vi "BioFeedback22(v_0.3).vi"() -> ()   [LabVIEW 2016]
doc: "Use this template to build a producer/consumer design pattern. Use this template when you need to execute a process, such as data analysis, when a data source, such as a triggered acquisition, produces data at an uneven rate and you need to execute the process when the data becomes available."
uses:
  customSubVIs/8ChanWfmArray.ctl
  <vilib>/Utility/file.llb/Write Delimited Spreadsheet (string).vi
panel:
  in  "infiniteTrial":bool=TRUE caption="Infinite Trial"
  out "MVC State":enum16{"Nothing", "Saved MVC", "NoSave MVC"}(ring)
  in  "MVC Delay (s)":dbl=3.0
  out "trial last time":timestamp
  out "mvc last time":timestamp
  in  "Display Width for MVC (s)":dbl(slide)=1.0 caption="Window Width in Seconds" scale=0.1..10.0
  in  "Display Width for Current Trial":dbl(slide)=1.0 caption="Window Width in Seconds" scale=0.1..10.0
  out "Current Trial (Filtered)":waveform(dbl)(graph)
  out "Current MVC (Filtered)":waveform(dbl)(graph)
  in  "enableSave":bool=TRUE caption="No Save      Save"
  in  "barOrGraph":bool=TRUE caption="Graph (under construction)       Bar"
  in  "Trial comment":string
  out "Collecting Data":bool
  in  "Display Min":dbl
  in  "Display Max":dbl=100.0
  in  "log filepath":path
  out "TrialStartTime":timestamp
  in  "Trial Duration (s)":dbl=3.0
  out "Trial Number":dbl
  in  "Session Name":string="Default"
  out "loopTime":dbl=30.0 caption="Upper Cut-Off"
  in  "trial display data":path
  out "Disp Data":cluster{"queue out":refnum<queue>, dbl, dbl}[](array[cluster])
  in  "Target Percentage":dbl=10.0
  out "Current Activation":dbl
  out "DisplayBarActivation":dbl(slide) caption="Percent Activation" max=1.0 scale=0.0..100.0
  in  "EMG Channel To Display":dbl=1.0
  out "MVC Data":cluster{"queue out":refnum<queue>, dbl, dbl}[](array[cluster])
  out "Trial Name":string="Test"
  in  "Data Directory":path=path "C:/Users/Tinggroup/Desktop/EMG Biofeedback System/LabviewFiles/Data"
  out "GetMaxStartTime":timestamp
  in  "MVC Number":dbl=3.0
  in  "MVC Duration (s)":dbl=3.0
  in  "Frames Per Second":dbl=30.0 caption="Upper Cut-Off"
  in  "EMG Input Device\nProduct Type":string="USB-6009"
  out "raw data":dynamicdata(graph)
  out "dispSize":dbl=20.0 caption="Lower Cut-Off"
  out "mvcSize":dbl=300.0 caption="Upper Cut-Off"
  in  "MVC Window Size (s)":dbl=0.5
  in  "Display Window Size (s)":dbl=0.5
  in  "MVC Raw Path":path
  in  "trial raw data":path
  in  "trial filtered data":path
  in  "MVC Filtered Path":path
  in  "Sample rate (Hz)":dbl=1000.0 caption="Upper Cut-Off"
  out "fps":dbl=20.0 caption="Lower Cut-Off"
  out "rate":dbl=300.0 caption="Upper Cut-Off"
  in  "Set Parameters":bool
  out "lower":dbl=20.0 caption="Lower Cut-Off"
  out "upper":dbl=300.0 caption="Upper Cut-Off"
  in  "Lower Cut-Off":dbl=20.0
  in  "Upper Cut-Off":dbl=500.0
  in  "Mark":bool
  in  "End Trial":bool
  in  "Get MVC":bool
  in  "StartTrial":bool
  out "State":T1(ring)
  out "FilteredAndRectified":waveform(dbl)[](graph) caption="Filtered\nand\nRectified"
  in  "stop":bool
  # "Behind The Scenes"
  # "Add trial comment\nBEFORE beginning trial"
  # "Timing"
  # "Display Settings"
  # "Filtering"
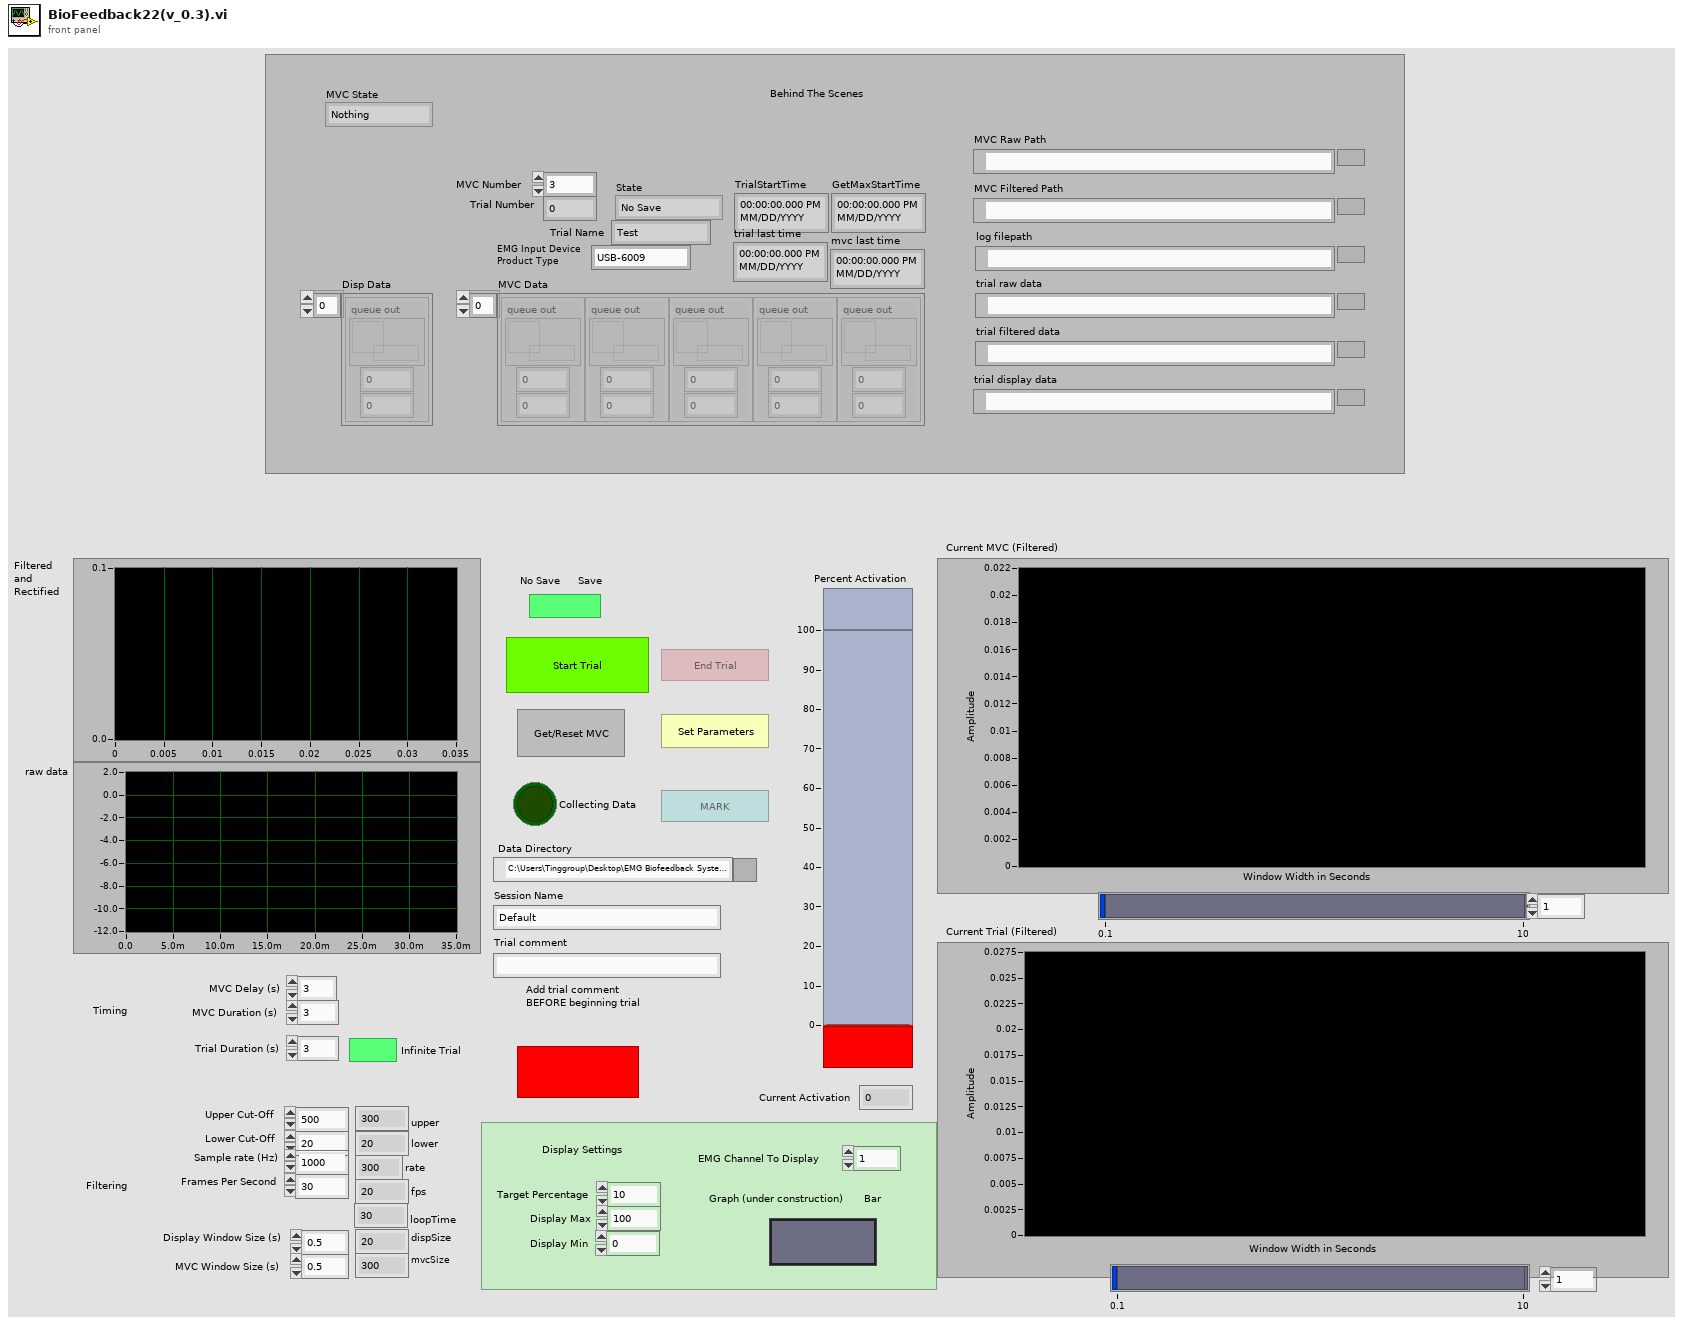
[diagram p1: front panel]
types:
  T1 = enum16{"No Save", "Acquiring Max", "Trial In Progress"}
  T2 = enum8{"Enabled", "Disabled", "Disabled and Grayed Out"}
  T3 = typedef "8ChanWfmArray.ctl" = waveform(dbl)[]
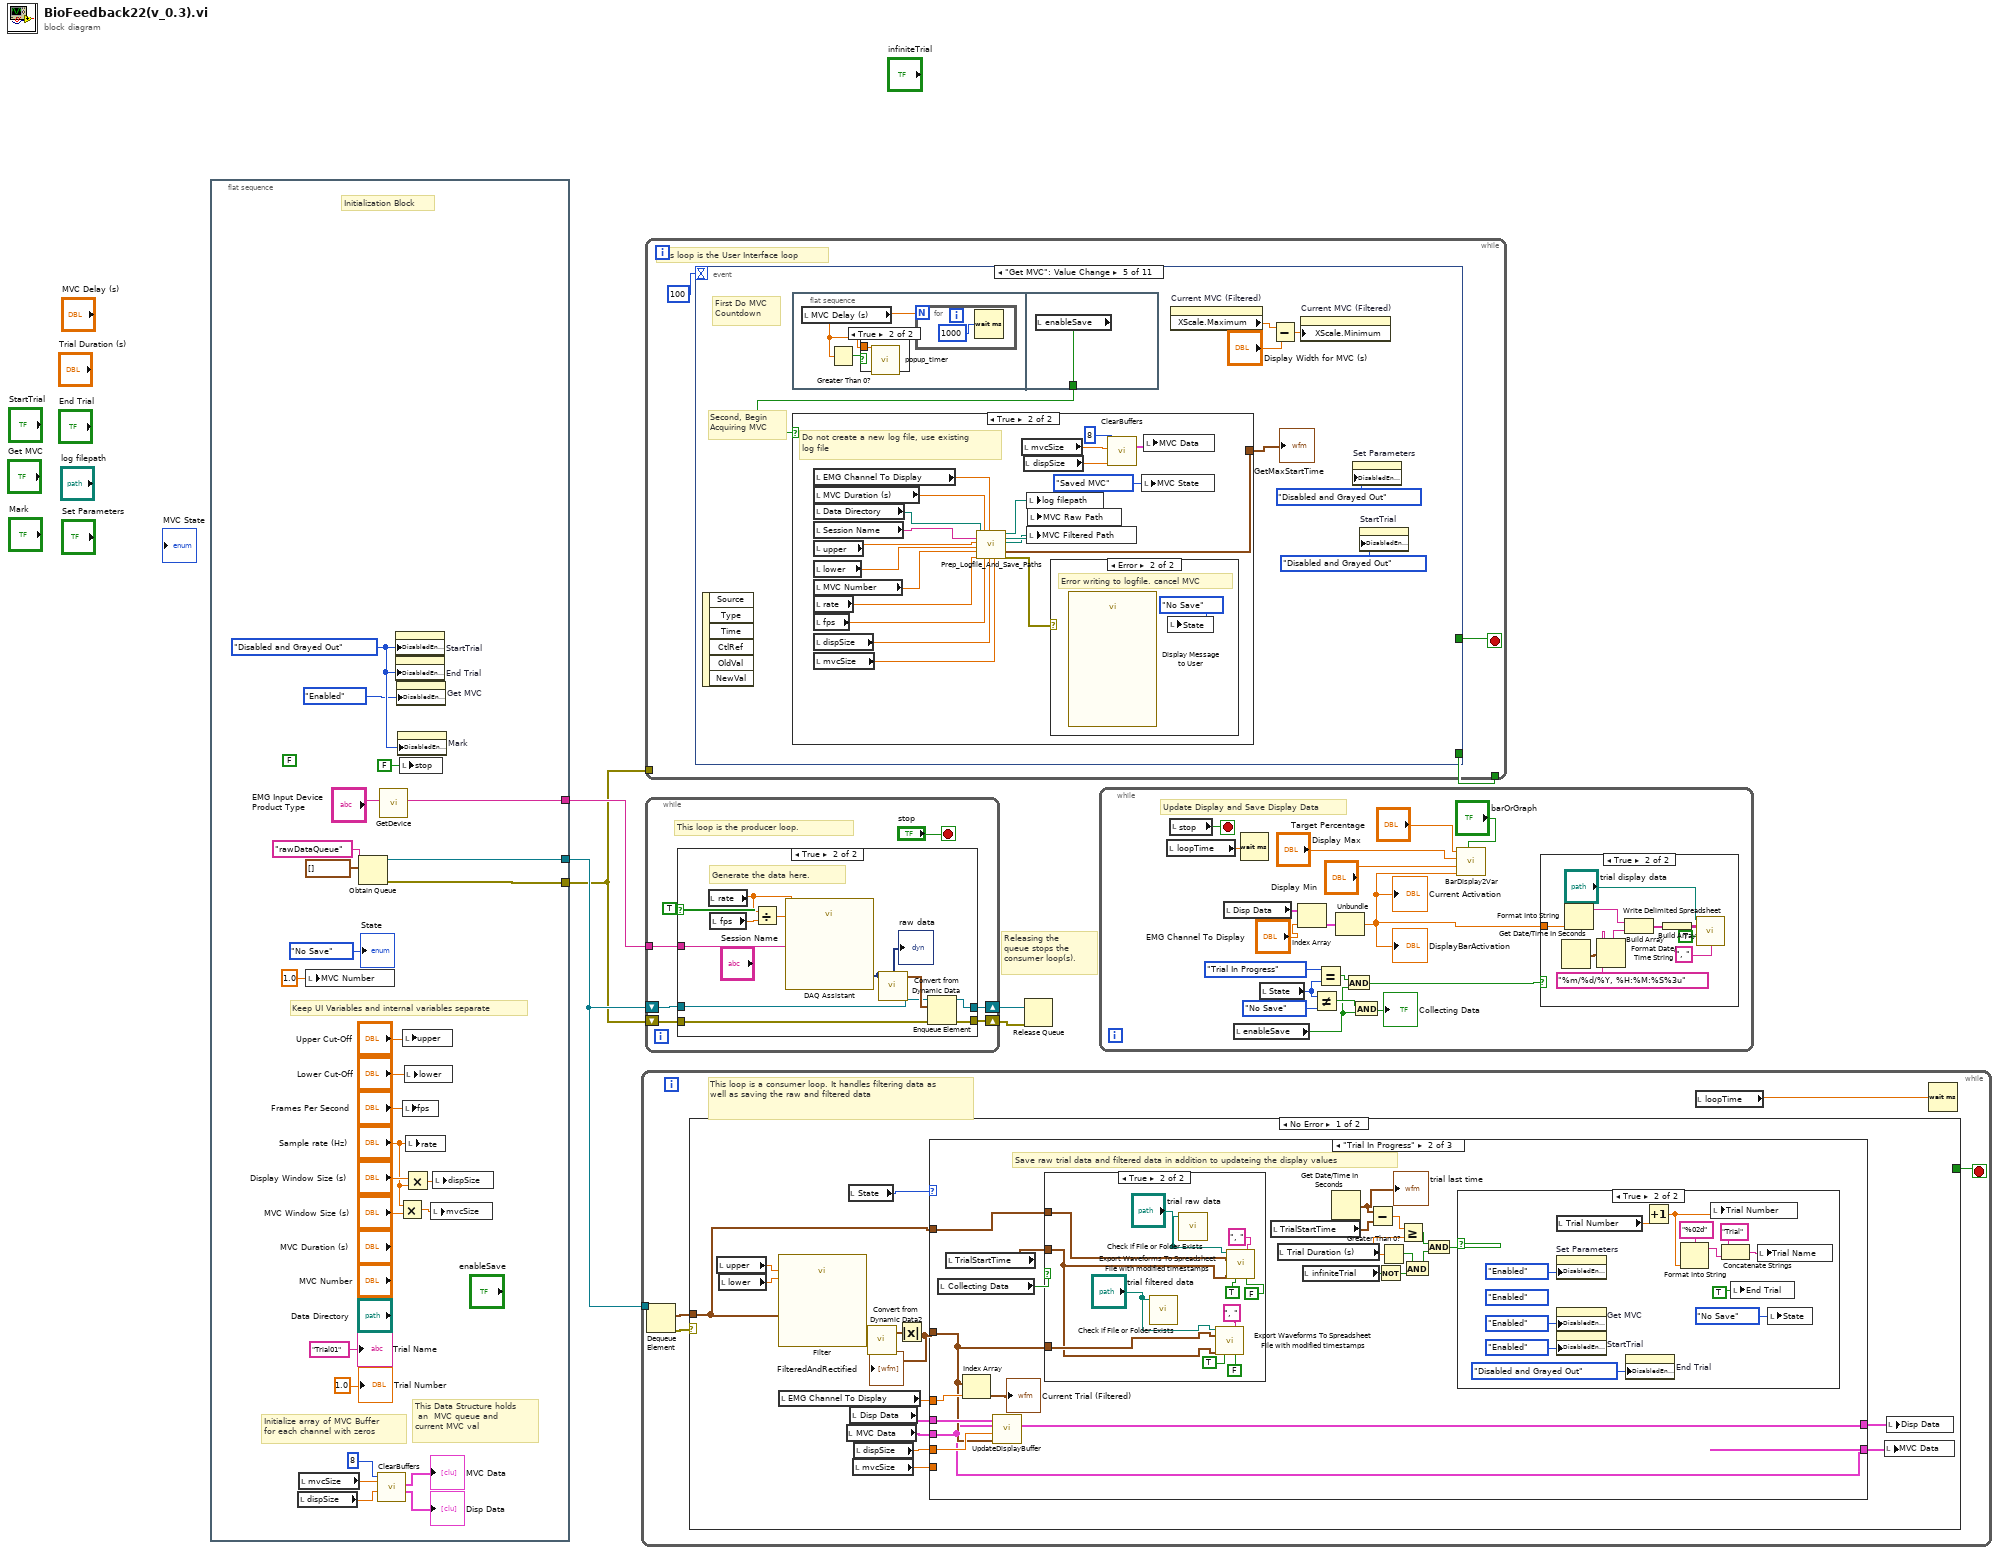
[diagram p0: block diagram]
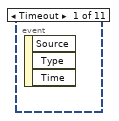
[diagram p3: hidden frame]
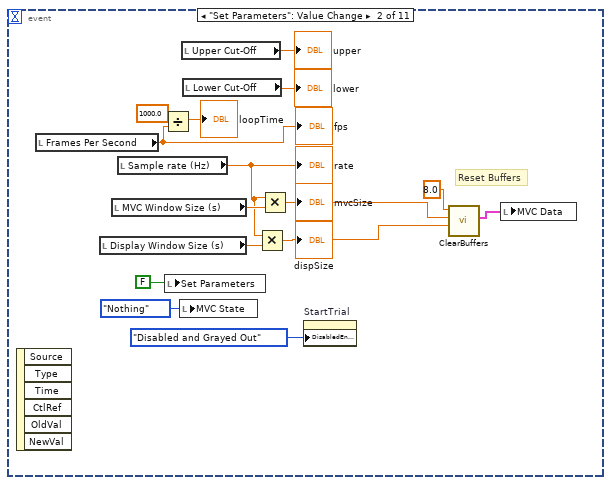
[diagram p4: hidden frame]
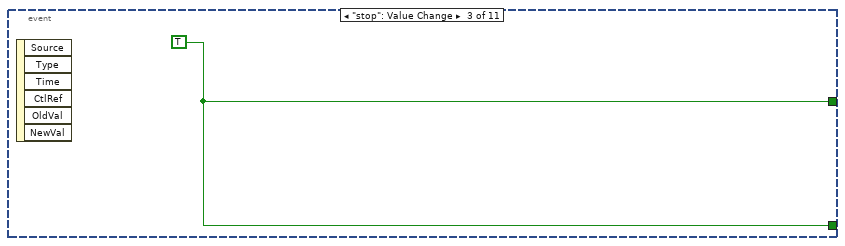
[diagram p5: hidden frame]
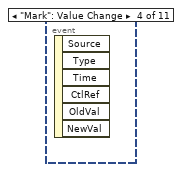
[diagram p6: hidden frame]
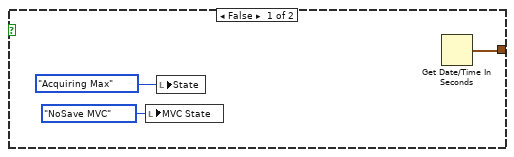
[diagram p8: hidden frame]
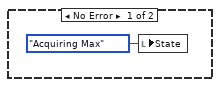
[diagram p9: hidden frame]
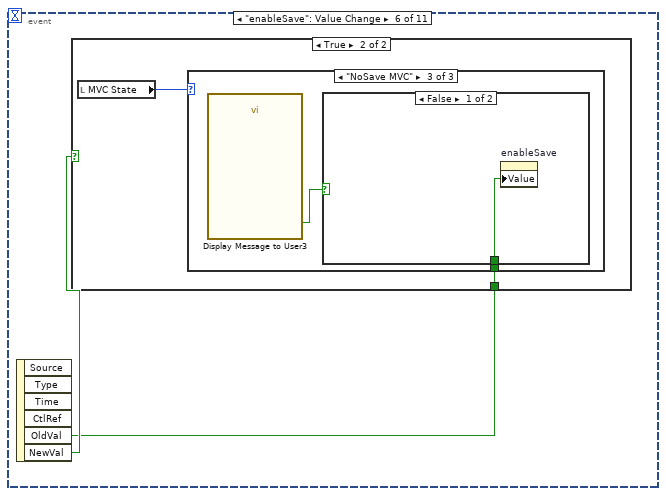
[diagram p10: hidden frame]
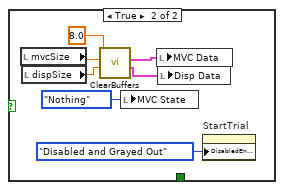
[diagram p14: hidden frame]
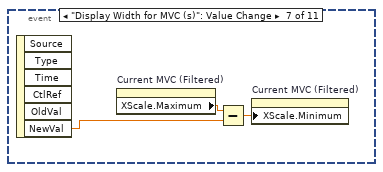
[diagram p15: hidden frame]
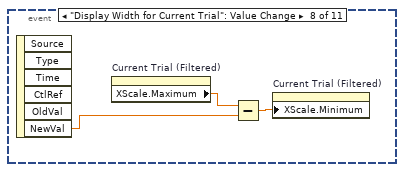
[diagram p16: hidden frame]
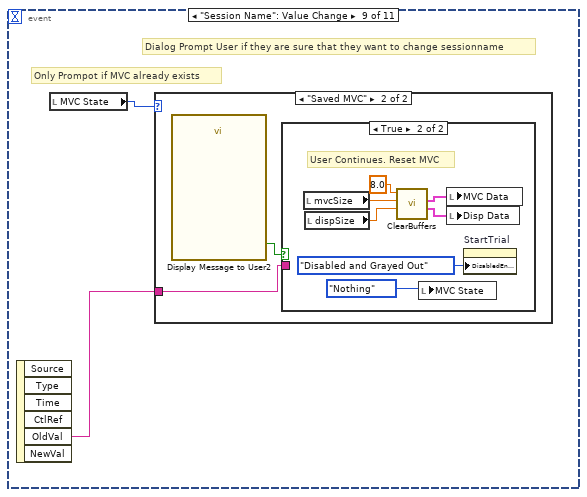
[diagram p17: hidden frame]
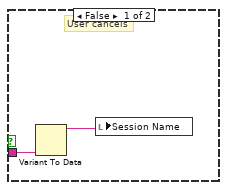
[diagram p19: hidden frame]
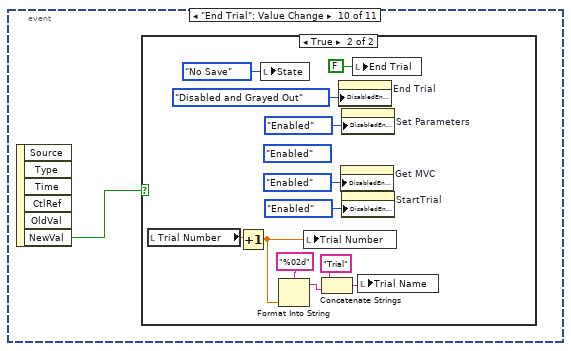
[diagram p20: hidden frame]
diagram:
  # "Releasing the\nqueue stops the consumer loop(s)."
  n1 = flat-sequence {
    tunnel: [w22] -> w2
    tunnel: [w21] -> w1
    tunnel: [w24] -> w3
    frame #0 {
      (unwired) FALSE ("Visible")
      w29 = T2."Disabled and Grayed Out" ("Disabled")
      # "Keep UI Variables and internal variables separate"
      # "This Data Structure holds\n an  MVC queue and \ncurrent MVC val"
      # "Initialize array of MVC Buffer \nfor each channel with zeros"
      # "Initialization Block"
      n2 = local read "dispSize"() -> (w9:dbl)
      n3 = local read "mvcSize"() -> (w10:dbl)
      n4 = local write "MVC Number"(1.0 ("MVC Number")) -> ()
      n5 = Obtain Queue(name (unnamed)="rawDataQueue", element data type=T3 [] ("initialized array")) -> (queue out=w22:refnum<queue>, error out=w21:errorcluster)  [unwired: 3 in, 1 out]
      n6 = call "ClearBuffers.vi"("disp size"=w9, "mvc size"=w10, "Num Channels"=8) -> ("Disp Data"=→"Disp Data":cluster{"queue out":refnum<queue>, dbl, dbl}[], "MVC Data"=→"MVC Data":cluster{"queue out":refnum<queue>, dbl, dbl}[])  [unwired: 7 in]
      n7 = call "GetDevice.vi"("EMG Input Device\nProduct Type"="EMG Input Device\nProduct Type") -> ("DAQmx Device Name"=w24:tag)  [unwired: 10 in]
      n8 = property on="StartTrial" class="Bool (strict)"("DisabledEnum"=w29) -> ()  [unwired: 2 in, 2 out]
      n9 = property on="End Trial" class="Bool (strict)"("DisabledEnum"=w29) -> ()  [unwired: 2 in, 2 out]
      n10 = property on="Get MVC" class="Bool"("DisabledEnum"=T2."Enabled" ("Disabled")) -> ()  [unwired: 2 in, 2 out]
      n11 = property on="Mark" class="Bool"("DisabledEnum"=w29) -> ()  [unwired: 2 in, 2 out]
      n12 = Multiply(x="Sample rate (Hz)", y="MVC Window Size (s)") -> (x*y=w16:dbl)
      n13 = local write "stop"(FALSE ("stop")) -> ()
      n14 = local write "upper"("Upper Cut-Off") -> ()
      n15 = local write "fps"("Frames Per Second") -> ()
      n16 = Multiply(x="Display Window Size (s)", y="Sample rate (Hz)") -> (x*y=w19:dbl)
      n17 = local write "lower"("Lower Cut-Off") -> ()
      n18 = local write "rate"("Sample rate (Hz)") -> ()
      n19 = local write "mvcSize"(w16) -> ()
      n20 = local write "dispSize"(w19) -> ()
      "Trial Name" <- "Trial01" ("Trial Name")
      "State" <- T1."No Save" ("State")
      "Trial Number" <- 1.0 ("Trial Number")
    }
  }
  n21 = while {
    tunnel: w2 -> [w33]
    stop <- w34 stop-if-true
    # "This loop is a consumer loop. It handles filtering data as well as saving the raw and filtered data"
    n22 = Dequeue Element(queue=w33) -> (element=w35:T3, error out=w36:errorcluster)  [unwired: 2 in, 2 out]
    n23 = case shown="No Error" w36 {
      tunnel: w35 -> [w46 _]
      tunnel: [_ TRUE] -> w34
      frame No Error {
        n24 = local read "upper"() -> (w48:dbl)
        n25 = local read "lower"() -> (w47:dbl)
        n26 = call "Filter"("Lower Cut-Off"=w47, "Upper Cut-Off"=w48, "Signal"=w46) -> ("Filtered Signal"=w49:dynamicdata)  [unwired: 7 in, 1 out]
        n27 = local read "EMG Channel To Display"() -> (w39:dbl)
        n28 = local read "MVC Data"() -> (w44:cluster{"queue out":refnum<queue>, dbl, dbl}[])
        n29 = local read "State"() -> (w40:T1)
        n30 = local read "Disp Data"() -> (w43:cluster{"queue out":refnum<queue>, dbl, dbl}[])
        n31 = local read "mvcSize"() -> (w37:dbl)
        n32 = local read "dispSize"() -> (w38:dbl)
        n33 = call "Convert from Dynamic Data2"("Dynamic Data Type"=w49) -> ("Array of Waveform"=w50:waveform(dbl)[])  [unwired: 3 in]
        n34 = Absolute Value(x=w50) -> (abs(x)=w45:waveform(dbl)[])
        "FilteredAndRectified" <- w45
        n35 = case shown="\"Trial In Progress\"" w40 {
          tunnel: w45 -> [w52 w61 w101]
          tunnel: w46 -> [_ w70 w110]
          tunnel: w44 -> [w54 w60 w104]
          tunnel: w43 -> [w55 w64 w105]
          tunnel: [w51 w62 w100] -> w41
          tunnel: [w54 w60 w99] -> w42
          tunnel: w39 -> [_ w67 w108]
          tunnel: w38 -> [w53 w63 w103]
          tunnel: w37 -> [_ _ w102]
          frame "No Save", Default {
            # "Update the display values, but do not save anything\n\nNote: MVC data is just referenced to calculate percent activation"
            n36 = call "UpdateDisplayBuffer.vi"("FilteredAndRectified"=w52, "dispSize"=w53, "MVC Data"=w54, "Disp Data"=w55) -> ("Disp Data Out"=w51:cluster{"queue out":refnum<queue>, dbl, dbl}[])  [unwired: 7 in]
          }
          frame "Trial In Progress" {
            # "Save raw trial data and filtered data in addition to updateing the display values"
            n37 = local read "Collecting Data"() -> (w69:bool)
            n38 = local read "TrialStartTime"() -> (w68:timestamp)
            n39 = Index Array(array=w61, index=w67) -> (element=→"Current Trial (Filtered)":waveform(dbl))
            n40 = call "UpdateDisplayBuffer.vi"("FilteredAndRectified"=w61, "dispSize"=w63, "MVC Data"=w60, "Disp Data"=w64) -> ("Disp Data Out"=w62:cluster{"queue out":refnum<queue>, dbl, dbl}[])  [unwired: 7 in]
            n41 = case shown="True" w69 {
              tunnel: w61 -> [_ w84]
              tunnel: w70 -> [_ w78]
              tunnel: w68 -> [_ w79]
              frame False {
              }
              frame True {
                n42 = call <vilib>:"Check if File or Folder Exists.vi"("path"="trial filtered data") -> ()  [unwired: 8 in, 3 out]
                n43 = call <vilib>:"Check if File or Folder Exists.vi"("path"="trial raw data") -> ()  [unwired: 8 in, 3 out]
                n44 = call "Export Waveforms To Spreadsheet File with modified timestamps.vi"("file path (dialog if empty)"="trial filtered data", "delimiter (Tab)"=", ", "waveforms"=w84, "trial start time"=w79, "append to file? (new file:F)"=TRUE, "header? (write header:T)"=FALSE) -> ()  [unwired: 8 in, 2 out]
                n45 = call "Export Waveforms To Spreadsheet File with modified timestamps.vi"("file path (dialog if empty)"="trial raw data", "delimiter (Tab)"=", ", "waveforms"=w78, "trial start time"=w79, "append to file? (new file:F)"=TRUE, "header? (write header:T)"=FALSE) -> ()  [unwired: 8 in, 2 out]
              }
            }
            n46 = local read "TrialStartTime"() -> (w74:timestamp)
            n47 = local read "Trial Duration (s)"() -> (w72:dbl)
            n48 = local read "infiniteTrial"() -> (w56:bool)
            n49 = Get Date/Time In Seconds() -> (seconds since 1Jan1904=w65:timestamp)
            "trial last time" <- w65
            n50 = Subtract(x=w65, y=w74) -> (x-y=w75:dbl)
            n51 = Not(x=w56) -> (.not. x?=w59:bool)
            n52 = Greater Than 0?(x=w72) -> (x > 0?=w58:bool)
            n53 = Greater Or Equal?(x=w75, y=w72) -> (x >= y?=w71:bool)
            n54 = And(x=w58, y=w59) -> (x .and. y?=w57:bool)
            n55 = And(x=w71, y=w57) -> (x .and. y?=w73:bool)
            n56 = case shown="True" w73 {
              frame False {
              }
              frame True {
                (unwired) T2."Enabled" ("Disabled")
                n57 = local read "Trial Number"() -> (w88:dbl)
                n58 = property on="Set Parameters" class="Bool (strict)"("DisabledEnum"=T2."Enabled" ("Disabled")) -> ()  [unwired: 2 in, 2 out]
                n59 = property on="Get MVC" class="Bool"("DisabledEnum"=T2."Enabled" ("Disabled")) -> ()  [unwired: 2 in, 2 out]
                n60 = property on="StartTrial" class="Bool (strict)"("DisabledEnum"=T2."Enabled" ("Disabled")) -> ()  [unwired: 2 in, 2 out]
                n61 = property on="End Trial" class="Bool (strict)"("DisabledEnum"=T2."Disabled and Grayed Out" ("Disabled")) -> ()  [unwired: 2 in, 2 out]
                n62 = Increment(x=w88) -> (x+1=w87:dbl)
                n63 = Format Into String(format string="%02d", w87) -> (resulting string=w93:string)  [unwired: 2 in, 1 out]
                n64 = local write "Trial Number"(w87) -> ()
                n65 = Concatenate Strings("Trial" ("string"), w93) -> (w97:string)
                n66 = local write "End Trial"(TRUE ("End Trial")) -> ()
                n67 = local write "Trial Name"(w97) -> ()
                n68 = local write "State"(T1."No Save" ("State")) -> ()
              }
            }
          }
          frame "Acquiring Max" {
            # "Automatically Stop Listening for Max after Acquire Max Time is elapsed"
            n69 = local read "GetMaxStartTime"() -> (w109:timestamp)
            n70 = local read "Collecting Data"() -> (w111:bool)
            n71 = call "UpdateMovingAverages.vi"("FilteredAndRectified"=w101, "mvcSize"=w102, "dispSize"=w103, "MVC Data"=w104, "Disp Data"=w105) -> ("MVC Data Out"=w99:cluster{"queue out":refnum<queue>, dbl, dbl}[], "Disp Data Out"=w100:cluster{"queue out":refnum<queue>, dbl, dbl}[])  [unwired: 5 in]
            n72 = case shown="True" w111 {
              tunnel: w110 -> [_ w118]
              tunnel: w101 -> [_ w124]
              tunnel: w109 -> [_ w119]
              frame False {
              }
              frame True {
                n73 = call "Export Waveforms To Spreadsheet File with modified timestamps.vi"("file path (dialog if empty)"="MVC Filtered Path", "delimiter (Tab)"=", ", "waveforms"=w124, "trial start time"=w119, "append to file? (new file:F)"=TRUE, "header? (write header:T)"=FALSE) -> ()  [unwired: 8 in, 2 out]
                n74 = call "Export Waveforms To Spreadsheet File with modified timestamps.vi"("file path (dialog if empty)"="MVC Raw Path", "delimiter (Tab)"=", ", "waveforms"=w118, "trial start time"=w119, "append to file? (new file:F)"=TRUE, "header? (write header:T)"=FALSE) -> ()  [unwired: 8 in, 2 out]
              }
            }
            n75 = Index Array(array=w101, index=w108) -> (element=→"Current MVC (Filtered)":waveform(dbl))
            n76 = local read "GetMaxStartTime"() -> (w115:timestamp)
            n77 = local read "MVC Duration (s)"() -> (w113:dbl)
            n78 = Get Date/Time In Seconds() -> (seconds since 1Jan1904=w106:timestamp)
            "mvc last time" <- w106
            n79 = Subtract(x=w106, y=w115) -> (x-y=w114:dbl)
            n80 = Greater Or Equal?(x=w114, y=w113) -> (x >= y?=w112:bool)
            n81 = case shown="True" w112 {
              frame False {
              }
              frame True {
                w128 = T2."Enabled" ("Disabled")
                n82 = local read "Collecting Data"() -> (w127:bool)
                n83 = local write "State"(T1."No Save" ("State")) -> ()
                n84 = property on="StartTrial" class="Bool (strict)"("DisabledEnum"=w128) -> ()  [unwired: 2 in, 2 out]
                n85 = property on="Set Parameters" class="Bool (strict)"("DisabledEnum"=w128) -> ()  [unwired: 2 in, 2 out]
                n86 = case shown="True" w127 {
                  frame False {
                  }
                  frame True {
                    n87 = local read "MVC Number"() -> (w131:dbl)
                    n88 = Increment(x=w131) -> (x+1=w130:dbl)
                    n89 = local write "MVC Number"(w130) -> ()
                  }
                }
              }
            }
          }
        }
        n90 = local write "MVC Data"(w42) -> ()
        n91 = local write "Disp Data"(w41) -> ()
      }
      frame Error {
        # "Return true for any case which should stop the loop."
      }
    }
    n92 = local read "loopTime"() -> (w32:dbl)
    n93 = Wait (ms)(milliseconds to wait=w32) -> ()  [unwired: 1 out]
  }
  n94 = while {
    tunnel: [w134] -> _
    tunnel: w1 -> [_]
    stop <- w133 stop-if-true
    # "This loop is the User Interface loop"
    n95 = event shown="[4] \"Get MVC\": Value Change" {
      selector: _ -> [_ _ _ _ _ _ _ _ _ _ _]
      dyn-events: _ -> [_ _ _ _ _ _ _ _ _ _ _]
      timeout: u32 100 ("milliseconds to wait") -> [_ _ _ _ _ _ _ _ _ _ _]
      tunnel: [_ _ w151 _ _ _ _ _ _ _ _] -> w133
      tunnel: [_ _ w151 _ _ _ _ _ _ _ _] -> w134
      event Timeout {
        n96 = event-data() -> ()  [unwired: 1 in, 3 out]
      }
      event "Set Parameters": Value Change {
        # "Reset Buffers"
        n97 = event-data() -> ()  [unwired: 1 in, 6 out]
        n98 = local read "Frames Per Second"() -> (w143:dbl)
        "fps" <- w143
        n99 = local read "Display Window Size (s)"() -> (w148:dbl)
        n100 = local read "MVC Window Size (s)"() -> (w149:dbl)
        n101 = local read "Sample rate (Hz)"() -> (w146:dbl)
        "rate" <- w146
        n102 = Divide(x=1000.0, y=w143) -> (x/y=→"loopTime":dbl)
        n103 = local write "Set Parameters"(FALSE ("Set Parameters")) -> ()
        n104 = local write "MVC State"(enum16{"Nothing", "Saved MVC", "NoSave MVC"}."Nothing" ("MVC State")) -> ()
        n105 = local read "Upper Cut-Off"() -> (→"upper":dbl)
        n106 = local read "Lower Cut-Off"() -> (→"lower":dbl)
        n107 = Multiply(x=w146, y=w148) -> (x*y=w140:dbl)
        "dispSize" <- w140
        n108 = Multiply(x=w146, y=w149) -> (x*y=w141:dbl)
        "mvcSize" <- w141
        n109 = property on="StartTrial" class="Bool (strict)"("DisabledEnum"=T2."Disabled and Grayed Out" ("Disabled")) -> ()  [unwired: 2 in, 2 out]
        n110 = call "ClearBuffers.vi"("disp size"=w140, "mvc size"=w141, "Num Channels"=8.0) -> ("MVC Data"=w138:cluster{"queue out":refnum<queue>, dbl, dbl}[])  [unwired: 7 in, 1 out]
        n111 = local write "MVC Data"(w138) -> ()
      }
      event "stop": Value Change {
        w151 = TRUE
        n112 = event-data() -> ()  [unwired: 1 in, 6 out]
      }
      event "Mark": Value Change {
        n113 = event-data() -> ()  [unwired: 1 in, 6 out]
      }
      event "Get MVC": Value Change {
        # "Second, Begin \nAcquiring MVC"
        # "First Do MVC\nCountdown"
        n114 = event-data() -> ()  [unwired: 1 in, 6 out]
        n115 = flat-sequence {
          tunnel: [w163] -> w156
          frame #0 {
            n116 = local read "MVC Delay (s)"() -> (w159:dbl)
            n117 = Greater Than 0?(x=w159) -> (x > 0?=w160:bool)
            n118 = case shown="True" w160 {
              tunnel: w159 -> [_ w161]
              frame False {
              }
              frame True {
                n119 = call "popup_timer.vi"("Seconds"=w161) -> ()  [unwired: 9 in, 1 out]
              }
            }
            n120 = for {
              N: w159 -> [_]
              n121 = Wait (ms)(milliseconds to wait=u32 1000) -> ()  [unwired: 1 out]
            }
          }
          frame #1 {
            n122 = local read "enableSave"() -> (w163:bool)
          }
        }
        n123 = case shown="True" w156 {
          tunnel: [w164 w167] -> w154
          frame False {
            n124 = local write "MVC State"(enum16{"Nothing", "Saved MVC", "NoSave MVC"}."NoSave MVC" ("MVC State")) -> ()
            n125 = local write "State"(T1."Acquiring Max" ("State")) -> ()
            n126 = Get Date/Time In Seconds() -> (seconds since 1Jan1904=w164:timestamp)
          }
          frame True {
            # "Do not create a new log file, use existing \nlog file"
            n127 = local read "EMG Channel To Display"() -> (w170:dbl)
            n128 = local read "MVC Duration (s)"() -> (w171:dbl)
            n129 = local read "Data Directory"() -> (w183:path)
            n130 = local read "Session Name"() -> (w182:string)
            n131 = local read "upper"() -> (w179:dbl)
            n132 = local read "lower"() -> (w178:dbl)
            n133 = local read "MVC Number"() -> (w177:dbl)
            n134 = local read "rate"() -> (w175:dbl)
            n135 = local read "fps"() -> (w174:dbl)
            n136 = local read "dispSize"() -> (w173:dbl)
            n137 = local read "mvcSize"() -> (w172:dbl)
            n138 = call "Prep_Logfile_And_Save_Paths.vi"("Data Directory"=w183, "Session Name"=w182, "upper"=w179, "lower"=w178, "MVC Number"=w177, "rate"=w175, "MVC Duration (s)"=w171, "fps"=w174, "EMG Channel To Display"=w170, "dispSize"=w173, "mvcSize"=w172) -> ("log filepath"=w181:path, "MVC Raw Path"=w180:path, "MVC Filtered Path"=w176:path, "GetMaxStartTime"=w167:timestamp, "error out"=w169:errorcluster)  [unwired: 4 in]
            n139 = local read "mvcSize"() -> (w186:dbl)
            n140 = local read "dispSize"() -> (w184:dbl)
            n141 = local write "log filepath"(w181) -> ()
            n142 = local write "MVC Filtered Path"(w176) -> ()
            n143 = local write "MVC Raw Path"(w180) -> ()
            n144 = case shown="Error" w169 {
              frame No Error {
                n145 = local write "State"(T1."Acquiring Max" ("State")) -> ()
              }
              frame Error {
                # "Error writing to logfile. cancel MVC"
                n146 = call "Display Message to User"() -> ()  [unwired: 10 in, 2 out]
                n147 = local write "State"(T1."No Save" ("State")) -> ()
              }
            }
            n148 = call "ClearBuffers.vi"("disp size"=w184, "mvc size"=w186, "Num Channels"=8) -> ("MVC Data"=w187:cluster{"queue out":refnum<queue>, dbl, dbl}[])  [unwired: 7 in, 1 out]
            n149 = local write "MVC State"(enum16{"Nothing", "Saved MVC", "NoSave MVC"}."Saved MVC" ("MVC State")) -> ()
            n150 = local write "MVC Data"(w187) -> ()
          }
        }
        "GetMaxStartTime" <- w154
        n151 = property on="Current MVC (Filtered)" class="WFChart (strict)"() -> ("XScale.Maximum"=w152:dbl)  [unwired: 2 in, 2 out]
        n152 = Subtract(x=w152, y="Display Width for MVC (s)") -> (x-y=w155:dbl)
        n153 = property on="Current MVC (Filtered)" class="WFChart (strict)"("XScale.Minimum"=w155) -> ()  [unwired: 2 in, 2 out]
        n154 = property on="Set Parameters" class="Bool (strict)"("DisabledEnum"=T2."Disabled and Grayed Out" ("Disabled")) -> ()  [unwired: 2 in, 2 out]
        n155 = property on="StartTrial" class="Bool (strict)"("DisabledEnum"=T2."Disabled and Grayed Out" ("Disabled")) -> ()  [unwired: 2 in, 2 out]
      }
      event "enableSave": Value Change {
        n156 = event-data() -> ("OldVal"=w190:bool, "NewVal"=w191:bool)  [unwired: 1 in, 4 out]
        n157 = case shown="True" w191 {
          tunnel: w190 -> [_ w192]
          frame False {
          }
          frame True {
            n158 = local read "MVC State"() -> (w193:enum16{"Nothing", "Saved MVC", "NoSave MVC"})
            n159 = case shown="\"NoSave MVC\"" w193 {
              tunnel: w192 -> [_ _ w194]
              frame "Nothing", Default {
              }
              frame "Saved MVC" {
              }
              frame "NoSave MVC" {
                n160 = call "Display Message to User3"() -> ("Enable Saving"=w195:bool)  [unwired: 10 in, 1 out]
                n161 = case shown="False" w195 {
                  tunnel: w194 -> [w196 _]
                  frame False {
                    n162 = property on="enableSave" class="Bool (strict)"("Value"=w196) -> ()  [unwired: 2 in, 2 out]
                  }
                  frame True {
                    n163 = local read "mvcSize"() -> (w201:dbl)
                    n164 = local read "dispSize"() -> (w200:dbl)
                    n165 = call "ClearBuffers.vi"("disp size"=w200, "mvc size"=w201, "Num Channels"=8.0) -> ("Disp Data"=w203:cluster{"queue out":refnum<queue>, dbl, dbl}[], "MVC Data"=w202:cluster{"queue out":refnum<queue>, dbl, dbl}[])  [unwired: 7 in]
                    n166 = local write "MVC State"(enum16{"Nothing", "Saved MVC", "NoSave MVC"}."Nothing" ("MVC State")) -> ()
                    n167 = local write "MVC Data"(w202) -> ()
                    n168 = local write "Disp Data"(w203) -> ()
                    n169 = property on="StartTrial" class="Bool (strict)"("DisabledEnum"=T2."Disabled and Grayed Out" ("Disabled")) -> ()  [unwired: 2 in, 2 out]
                  }
                }
              }
            }
          }
        }
      }
      event "Display Width for MVC (s)": Value Change {
        n170 = event-data() -> ("NewVal"=w206:dbl)  [unwired: 1 in, 5 out]
        n171 = property on="Current MVC (Filtered)" class="WFChart (strict)"() -> ("XScale.Maximum"=w204:dbl)  [unwired: 2 in, 2 out]
        n172 = Subtract(x=w204, y=w206) -> (x-y=w205:dbl)
        n173 = property on="Current MVC (Filtered)" class="WFChart (strict)"("XScale.Minimum"=w205) -> ()  [unwired: 2 in, 2 out]
      }
      event "Display Width for Current Trial": Value Change {
        n174 = event-data() -> ("NewVal"=w209:dbl)  [unwired: 1 in, 5 out]
        n175 = property on="Current Trial (Filtered)" class="WFChart (strict)"() -> ("XScale.Maximum"=w207:dbl)  [unwired: 2 in, 2 out]
        n176 = Subtract(x=w207, y=w209) -> (x-y=w208:dbl)
        n177 = property on="Current Trial (Filtered)" class="WFChart (strict)"("XScale.Minimum"=w208) -> ()  [unwired: 2 in, 2 out]
      }
      event "Session Name": Value Change {
        # "Only Prompot if MVC already exists"
        # "Dialog Prompt User if they are sure that they want to change sessionname"
        n178 = event-data() -> ("OldVal"=w211:string)  [unwired: 1 in, 5 out]
        n179 = local read "MVC State"() -> (w210:enum16{"Nothing", "Saved MVC", "NoSave MVC"})
        n180 = case shown="\"Saved MVC\"" w210 {
          tunnel: w211 -> [_ w212]
          frame "Nothing", Default {
          }
          frame "Saved MVC" {
            n181 = call "Display Message to User2"() -> ("Change"=w213:bool)  [unwired: 10 in, 1 out]
            n182 = case shown="True" w213 {
              tunnel: w212 -> [w215 _]
              frame False {
                # "User cancels"
                n183 = Variant To Data(Variant=w215) -> (data=w214:string)  [unwired: 2 in, 1 out]
                n184 = local write "Session Name"(w214) -> ()
              }
              frame True {
                # "User Continues. Reset MVC"
                n185 = local read "mvcSize"() -> (w221:dbl)
                n186 = local read "dispSize"() -> (w220:dbl)
                n187 = call "ClearBuffers.vi"("disp size"=w220, "mvc size"=w221, "Num Channels"=8.0) -> ("Disp Data"=w217:cluster{"queue out":refnum<queue>, dbl, dbl}[], "MVC Data"=w218:cluster{"queue out":refnum<queue>, dbl, dbl}[])  [unwired: 7 in]
                n188 = local write "MVC State"(enum16{"Nothing", "Saved MVC", "NoSave MVC"}."Nothing" ("MVC State")) -> ()
                n189 = local write "MVC Data"(w218) -> ()
                n190 = local write "Disp Data"(w217) -> ()
                n191 = property on="StartTrial" class="Bool (strict)"("DisabledEnum"=T2."Disabled and Grayed Out" ("Disabled")) -> ()  [unwired: 2 in, 2 out]
              }
            }
          }
        }
      }
      event "End Trial": Value Change {
        n192 = event-data() -> ("NewVal"=w223:bool)  [unwired: 1 in, 5 out]
        n193 = case shown="True" w223 {
          frame False {
          }
          frame True {
            (unwired) T2."Enabled" ("Disabled")
            n194 = local read "Trial Number"() -> (w228:dbl)
            n195 = Increment(x=w228) -> (x+1=w224:dbl)
            n196 = local write "State"(T1."No Save" ("State")) -> ()
            n197 = Format Into String(format string="%02d", w224) -> (resulting string=w227:string)  [unwired: 2 in, 1 out]
            n198 = local write "Trial Number"(w224) -> ()
            n199 = Concatenate Strings("Trial" ("string"), w227) -> (w229:string)
            n200 = property on="End Trial" class="Bool (strict)"("DisabledEnum"=T2."Disabled and Grayed Out" ("Disabled")) -> ()  [unwired: 2 in, 2 out]
            n201 = property on="Get MVC" class="Bool"("DisabledEnum"=T2."Enabled" ("Disabled")) -> ()  [unwired: 2 in, 2 out]
            n202 = property on="Set Parameters" class="Bool (strict)"("DisabledEnum"=T2."Enabled" ("Disabled")) -> ()  [unwired: 2 in, 2 out]
            n203 = property on="StartTrial" class="Bool (strict)"("DisabledEnum"=T2."Enabled" ("Disabled")) -> ()  [unwired: 2 in, 2 out]
            n204 = local write "End Trial"(FALSE ("End Trial")) -> ()
            n205 = local write "Trial Name"(w229) -> ()
          }
        }
      }
      event "StartTrial": Value Change {
        n206 = event-data() -> ("NewVal"=w236:bool)  [unwired: 1 in, 5 out]
        n207 = case shown="True" w236 {
          frame False {
          }
          frame True {
            (unwired) T2."Disabled and Grayed Out" ("Disabled")
            n208 = local write "StartTrial"(FALSE ("StartTrial")) -> ()
            n209 = local read "Data Directory"() -> (w284:path)
            n210 = local write "End Trial"(FALSE ("End Trial")) -> ()
            n211 = local read "Session Name"() -> (w283:string)
            n212 = local read "Trial Name"() -> (w268:string)
            n213 = local write "State"(T1."Trial In Progress" ("State")) -> ()
            n214 = Concatenate Strings(w268, "_FilteredData.csv" ("string")) -> (w288:string)
            n215 = Concatenate Strings(w268, "_RawData.csv" ("string")) -> (w286:string)
            n216 = Concatenate Strings(w268, "_DisplayData.csv" ("string")) -> (w290:string)
            n217 = property on="Current Trial (Filtered)" class="WFChart (strict)"() -> ("XScale.Maximum"=w237:dbl)  [unwired: 2 in, 2 out]
            n218 = Build Path(base path=w284, name or relative path=w283) -> (appended path=w267:path)
            n219 = property on="End Trial" class="Bool (strict)"("DisabledEnum"=T2."Enabled" ("Disabled")) -> ()  [unwired: 2 in, 2 out]
            n220 = property on="StartTrial" class="Bool (strict)"("DisabledEnum"=T2."Disabled and Grayed Out" ("Disabled")) -> ()  [unwired: 2 in, 2 out]
            n221 = property on="Get MVC" class="Bool"("DisabledEnum"=T2."Disabled and Grayed Out" ("Disabled")) -> ()  [unwired: 2 in, 2 out]
            n222 = property on="Set Parameters" class="Bool (strict)"("DisabledEnum"=T2."Disabled and Grayed Out" ("Disabled")) -> ()  [unwired: 2 in, 2 out]
            n223 = Build Path(base path=w267, name or relative path="Log.csv" ("string")) -> (appended path=w251:path)
            n224 = Build Path(base path=w267, name or relative path=w288) -> (appended path=w282:path)
            n225 = Build Path(base path=w267, name or relative path=w286) -> (appended path=w281:path)
            n226 = Build Path(base path=w267, name or relative path=w290) -> (appended path=w291:path)
            n227 = Get Date/Time In Seconds() -> (seconds since 1Jan1904=→"TrialStartTime":timestamp)
            n228 = local write "trial raw data"(w281) -> ()
            n229 = local write "log filepath"(w251) -> ()
            n230 = local write "trial filtered data"(w282) -> ()
            n231 = local write "trial display data"(w291) -> ()
            n232 = Subtract(x=w237, y="Display Width for Current Trial") -> (x-y=w240:dbl)
            n233 = property on="Current MVC (Filtered)" class="WFChart (strict)"("XScale.Minimum"=w240) -> ()  [unwired: 2 in, 2 out]
            n234 = local read "EMG Channel To Display"() -> (w247:dbl)
            n235 = local read "EMG Channel To Display"() -> (w277:dbl)
            n236 = local read "MVC Data"() -> (w248:cluster{"queue out":refnum<queue>, dbl, dbl}[])
            n237 = local read "MVC Duration (s)"() -> (w276:dbl)
            n238 = local read "dispSize"() -> (w274:dbl)
            n239 = local read "lower"() -> (w271:dbl)
            n240 = Index Array(array=w248, index=w247) -> (element=w246:cluster{"queue out":refnum<queue>, dbl, dbl})
            n241 = local read "mvcSize"() -> (w275:dbl)
            n242 = local read "upper"() -> (w270:dbl)
            n243 = local read "Trial Name"() -> (w264:string)
            n244 = local read "rate"() -> (w272:dbl)
            n245 = local read "fps"() -> (w273:dbl)
            n246 = Number To Decimal String(number=w271) -> (decimal integer string=w260:string)  [unwired: 1 in]
            n247 = Number To Decimal String(number=w274) -> (decimal integer string=w258:string)  [unwired: 1 in]
            n248 = Unbundle(w246) -> (w242:dbl)  [unwired: 2 out]
            n249 = Number To Decimal String(number=w277) -> (decimal integer string=w255:string)  [unwired: 1 in]
            n250 = Get Date/Time In Seconds() -> (seconds since 1Jan1904=w250:timestamp)
            n251 = Number To Decimal String(number=w270) -> (decimal integer string=w261:string)  [unwired: 1 in]
            n252 = Number To Decimal String(number=w272) -> (decimal integer string=w259:string)  [unwired: 1 in]
            n253 = Number To Decimal String(number=w273) -> (decimal integer string=w254:string)  [unwired: 1 in]
            n254 = Number To Decimal String(number=w275) -> (decimal integer string=w257:string)  [unwired: 1 in]
            n255 = Number To Decimal String(number=w276) -> (decimal integer string=w256:string)  [unwired: 1 in]
            n256 = Format Date/Time String(time format string (%c)="%m/%d/%Y %H:%M:%S%3u", seconds (now)=w250) -> (date/time string=w245:string)  [unwired: 1 in]
            n257 = Format Value(format string="%5f", value (0)=w242) -> (output string=w241:string)  [unwired: 1 in]
            n258 = Build Array(w264, w261, w260, w259, w254, w258, w257, w256, w255, w241, w245, "Trial comment") -> (w253:string[])
            n259 = call-poly <vilib>:"Write Delimited Spreadsheet.vi"("file path (dialog if empty)"=w251, "1D data"=w253, "append to file? (new file:F)"=TRUE, "delimiter (\\t)"=", " ("delimiter (\\t)")) -> ()  [unwired: 10 in, 2 out]
          }
        }
      }
    }
  }
  n260 = while {
    shift-right: [w296] -> w4
    shift-left: w1 -> [w297]
    shift-right: [w293] -> w5
    shift-left: w2 -> [w298]
    tunnel: w3 -> [w294]
    stop <- "stop" stop-if-true
    # "This loop is the producer loop."
    n261 = case shown="True" TRUE ("Case Constant\n(See Context Help)") {
      tunnel: w298 -> [w300 w303]
      tunnel: w297 -> [w301 w311]
      tunnel: [w301 w310] -> w296
      tunnel: w294 -> [_ w305]
      tunnel: [w300 w302] -> w293
      frame False {
      }
      frame True {
        # "Generate the data here."
        n262 = local read "rate"() -> (w308:dbl)
        n263 = local read "fps"() -> (w309:dbl)
        n264 = Divide(x=w308, y=w309) -> (x/y=w307:dbl)
        n265 = call "DAQ Assistant"("rate"=w308, "number of samples"=w307, "device name"=w305) -> ("data"=w306:dynamicdata)  [unwired: 13 in, 3 out]
        "raw data" <- w306
        n266 = call "Convert from Dynamic Data"("Dynamic Data Type"=w306) -> ("Array of Waveform"=w304:waveform(dbl)[])  [unwired: 3 in]
        n267 = Enqueue Element(queue=w303, element=w304, error in (no error)=w311) -> (queue out=w302:refnum<queue>, error out=w310:errorcluster)  [unwired: 1 in, 1 out]
      }
    }
  }
  n268 = Release Queue(queue=w5, error in (no error)=w4) -> ()  [unwired: 1 in, 3 out]
  n269 = while {
    stop <- w325 stop-if-true
    # "Update Display and Save Display Data"
    n270 = local read "loopTime"() -> (w324:dbl)
    n271 = local read "stop"() -> (w325:bool)
    n272 = local read "Disp Data"() -> (w328:cluster{"queue out":refnum<queue>, dbl, dbl}[])
    n273 = local read "enableSave"() -> (w315:bool)
    n274 = Wait (ms)(milliseconds to wait=w324) -> ()  [unwired: 1 out]
    n275 = local read "State"() -> (w316:T1)
    n276 = Index Array(array=w328, index="EMG Channel To Display") -> (element=w326:cluster{"queue out":refnum<queue>, dbl, dbl})
    n277 = Not Equal?(x=w316, y=T1."No Save" ("State")) -> (x != y?=w319:bool)
    n278 = Equal?(x=T1."Trial In Progress" ("State"), y=w316) -> (x = y?=w314:bool)
    n279 = Unbundle(w326) -> (w313:dbl)  [unwired: 2 out]
    "DisplayBarActivation" <- w313
    "Current Activation" <- w313
    n280 = And(x=w314, y=w315) -> (x .and. y?=w312:bool)
    n281 = And(x=w319, y=w315) -> (x .and. y?=→"Collecting Data":bool)
    n282 = call "BarDisplay2Var.vi"("barOrGraph"="barOrGraph", "Activation Percentage"=w313, "scale min"="Display Min", "scale max"="Display Max", "Target Percentage"="Target Percentage") -> ()  [unwired: 7 in]
    n283 = case shown="True" w312 {
      tunnel: w313 -> [_ w330]
      frame False {
      }
      frame True {
        n284 = Get Date/Time In Seconds() -> (seconds since 1Jan1904=w333:timestamp)
        n285 = Format Into String(w330) -> (resulting string=w335:string)  [unwired: 3 in, 1 out]
        n286 = Format Date/Time String(time format string (%c)="%m/%d/%Y, %H:%M:%S%3u", seconds (now)=w333) -> (date/time string=w334:string)  [unwired: 1 in]
        n287 = Build Array(w335, w334) -> (w336:string[])
        n288 = Build Array(w336) -> (w337:string[][])
        n289 = call-poly <vilib>:"Write Delimited Spreadsheet.vi"("file path (dialog if empty)"="trial display data", "2D data"=w337, "append to file? (new file:F)"=TRUE, "delimiter (\\t)"=", " ("delimiter (\\t)")) -> ()  [unwired: 10 in, 2 out]
      }
    }
  }
